vi "Read csv file.vi"() -> ()   [LabVIEW 2019]
uses:
  Support Code/Controls/Auto Controls.ctl
  <vilib>/Utility/file.llb/Read Delimited Spreadsheet (DBL).vi
panel:
  in  "index":i32
  out "Ring Text.Text":string
  out "File Recorded":T1(ring)
  out "Auto Commands":T2[](array[typedef])
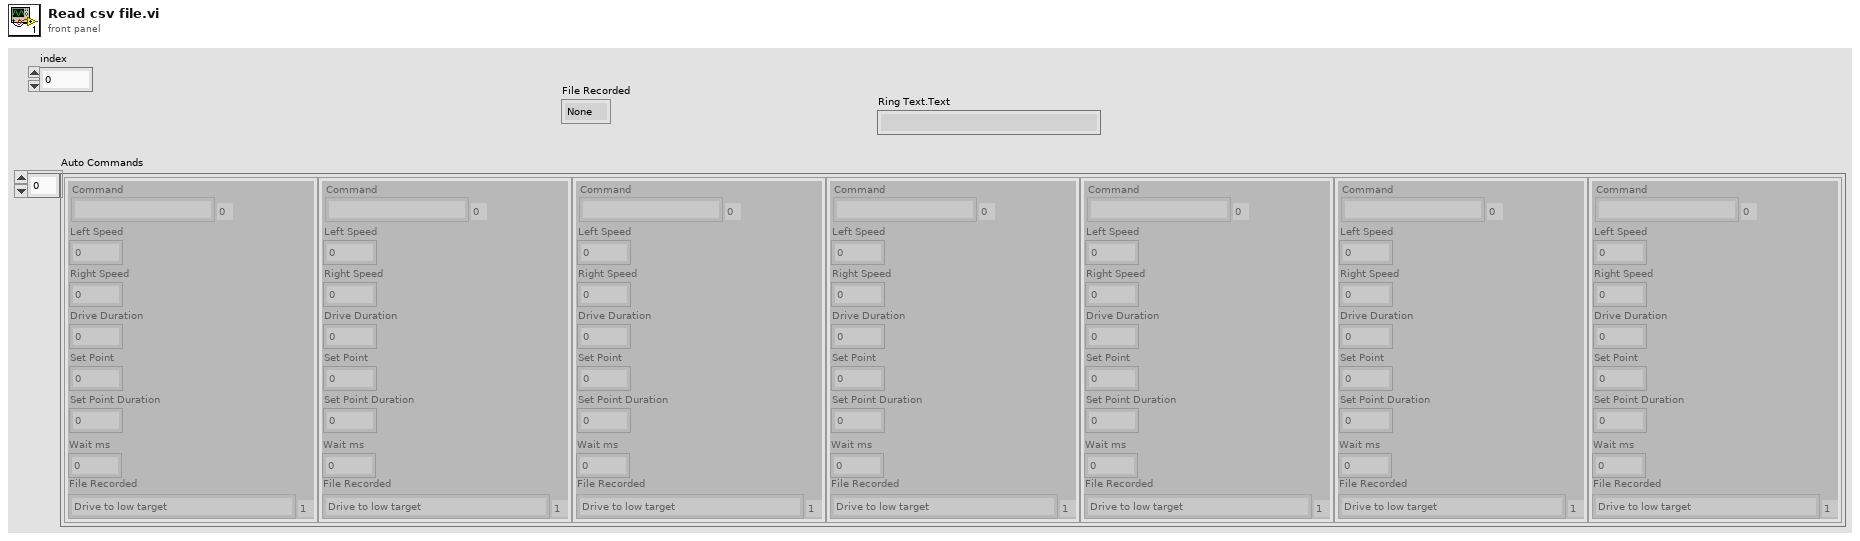
[diagram p1: front panel]
types:
  T1 = enum16{"None", "Drive to low target", "Drive to pick balls from the right CP", "Drive to pick up balls from the Left CP", "Drive to pick up 3 balls from the center", "Drive to pick up 2 balls from the center"}
  T2 = typedef "Auto Controls.ctl" = cluster{"Drive Duration":dbl, "Left Speed":dbl, "Right Speed":dbl, "Set Point":dbl, "Set Point Duration":dbl, "Command":enum16{"", "Drive Forwards", "Drive Backwards", "Stop", "Turn Left", "Turn Right", "Drop Intake", "Lift Intake", "Intake", "Shooter", "Transfer", "Wait", "Drive from recorded file"}, "Wait ms":dbl, "File Recorded":enum16{"None", "Drive to low target", "Drive to pick balls from the right CP", "Drive to pick up balls from the Left CP", "Drive to pick up 3 balls from the center", "Drive to pick up 2 balls from the center"}}
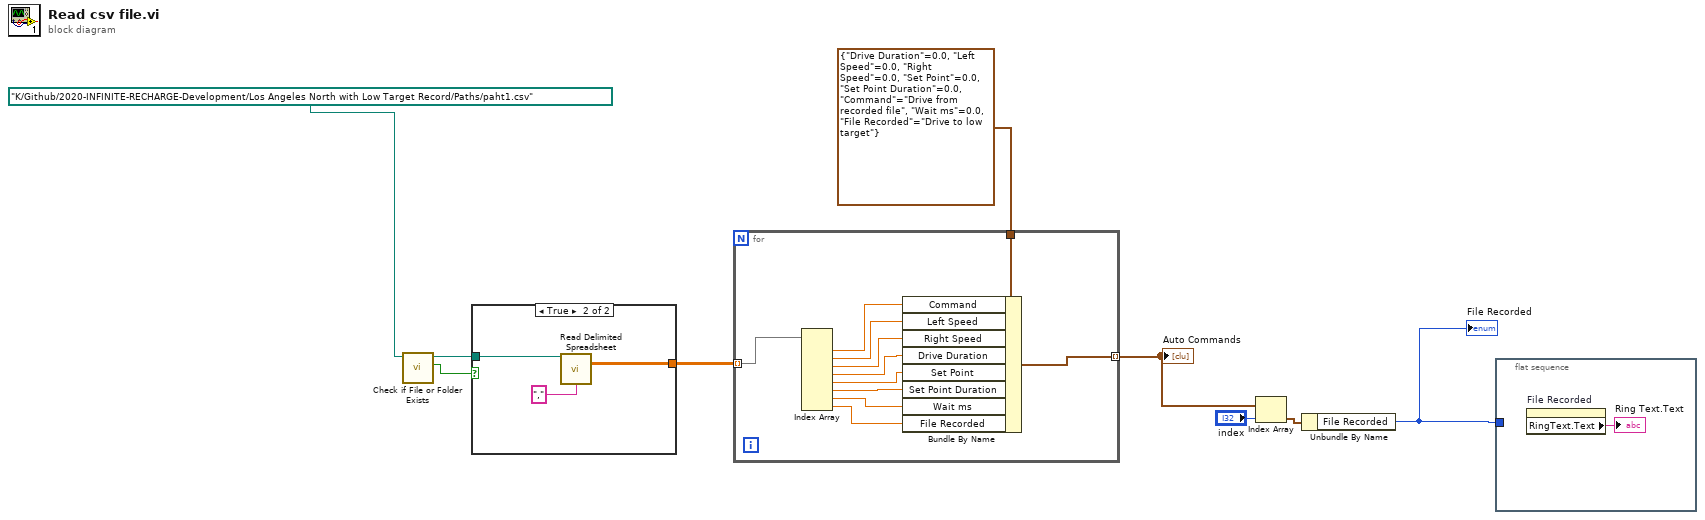
[diagram p0: block diagram]
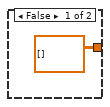
[diagram p2: hidden frame]
diagram:
  n1 = call <vilib>:"Check if File or Folder Exists.vi"("path"=path "K:/Github/2020-INFINITE-RECHARGE-Development/Los Angeles North with Low Target Record/Paths/paht1.csv") -> ("file or folder exists?"=w9:bool, "dup path"=w8:path)  [unwired: 8 in, 1 out]
  n2 = case shown="True" w9 {
    tunnel: w8 -> [_ w13]
    tunnel: [dbl[][] [] ("all rows") w11] -> w6
    frame False {
    }
    frame True {
      n3 = call-poly <vilib>:"Read Delimited Spreadsheet.vi"("file path (dialog if empty)"=w13, "delimiter (\\t)"="," ("delimiter (\\t)")) -> ("all rows"=w11:dbl[][])  [unwired: 8 in, 5 out]
    }
  }
  n4 = for {
    tunnel: T2 {"Drive Duration"=0.0, "Left Speed"=0.0, "Right Speed"=0.0, "Set Point"=0.0, "Set Point Duration"=0.0, "Command"=enum."Drive from recorded file", "Wait ms"=0.0, "File Recorded"=enum."Drive to low target"} ("Auto Control") -> [w24]
    tunnel: [w16] -> w4 mode=indexing
    tunnel: w6 -> [w15] mode=indexing
    n5 = Index Array(array=w15) -> (element #1=w23:dbl, element #2=w22:dbl, element #3=w21:dbl, element #4=w20:dbl, element #5=w19:dbl, element #6=w18:dbl, element #7=w17:dbl, element #8=w14:dbl)  [unwired: 8 in]
    n6 = Bundle By Name(cluster=w24, "Command"=w23, "Left Speed"=w22, "Right Speed"=w21, "Drive Duration"=w20, "Set Point"=w19, "Set Point Duration"=w18, "Wait ms"=w17, "File Recorded"=w14) -> (w16:T2)
  }
  "Auto Commands" <- w4
  n7 = Index Array(array=w4, index="index") -> (element=w3:T2)
  n8 = Unbundle By Name(w3) -> ("File Recorded"=w2:T1)
  "File Recorded" <- w2
  n9 = flat-sequence {
    tunnel: w2 -> [_]
    frame #0 {
      n10 = property on="File Recorded" class="Enum (strict)"() -> ("RingText.Text"=→"Ring Text.Text":string)  [unwired: 2 in, 2 out]
    }
  }
